vi "GetPropertyDefinitionFolders.vi"(8 "error in (no error)":errorcluster, 11 "ClassReflector in":refnum<class "ClassReflector.lvclass">) -> (0 "error out":errorcluster, 2 "PropertyDefinitionFolders":refnum<vi>[](array[refnum]), 3 "ClassReflector out":refnum<class "ClassReflector.lvclass">)   [LabVIEW 2023, in "ClassReflector.lvclass"]
uses:
  ClassReflector.lvclass
  ClassReflector.lvclass/ClassReflector.ctl
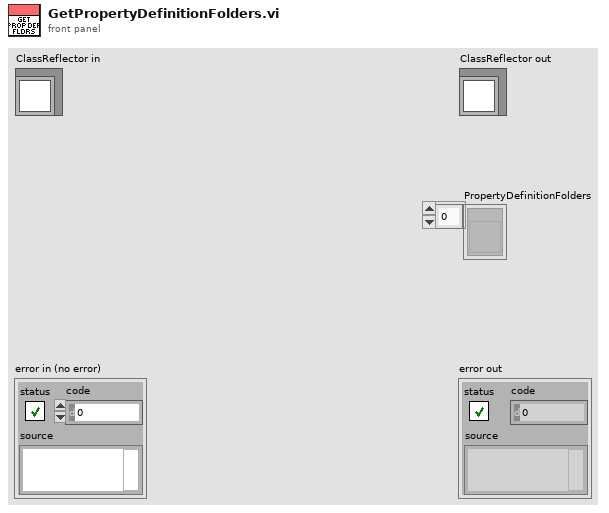
[diagram p1: front panel]
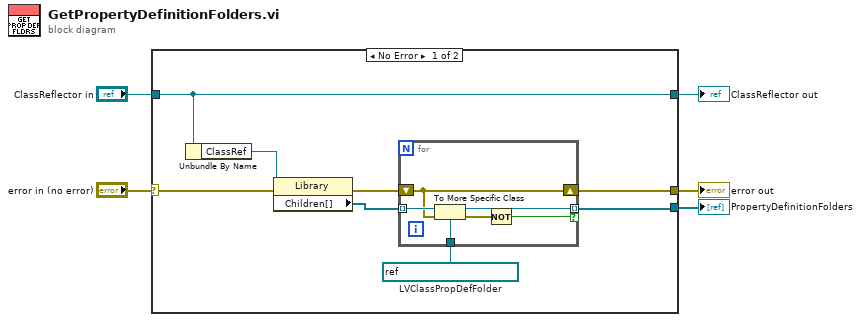
[diagram p0: block diagram]
diagram:
  n1 = case shown="No Error" "error in (no error)" {
    selector: "error in (no error)" -> [w10 w21]
    tunnel: [w6 w21] -> w4
    tunnel: [w13 w20] -> w2
    tunnel: "ClassReflector in" -> [w13 w20]
    tunnel: [w9 _] -> w1
    frame No Error {
      w11 = refnum<vi> refnum  # LVClassPropDefFolder
      n2 = Unbundle By Name(w13) -> ("ClassRef"=w12:refnum<vi>)
      n3 = property class="Library"(reference=w12, error in=w10) -> (error out=w8:errorcluster, "Children[]"=w7:refnum<vi>[])  [unwired: 1 out]
      n4 = for {
        tunnel: w11 -> [w19]
        tunnel: w7 -> [w18] mode=indexing
        tunnel: [w17] -> w9 mode=indexing if=w14
        shift-right: [w16] -> w6
        shift-left: w8 -> [w16]
        n5 = To More Specific Class(target class=w19, reference=w18, error in=w16) -> (specific class reference=w17:refnum<vi>, error out=w15:errorcluster)
        n6 = Not(x=w15) -> (.not. x?=w14:bool)
      }
    }
    frame Error {
    }
  }
  "error out" <- w4
  "ClassReflector out" <- w2
  "PropertyDefinitionFolders" <- w1
